vi "DequeueMessage.vi"(8 "error in (no error)":errorcluster, 9 "ms timeout (-1)":i32=-1, 11 "queue in":refnum<data-value>) -> (0 "error out":errorcluster, 1 "timeout":bool, 2 "message":variant, 3 "queue out":refnum<data-value>)   [LabVIEW 2009, in "PriorityQueue.lvclass"]
uses:
  PriorityQueue.lvclass
  LinkedList/position.ctl
  PriorityQueue.lvclass/PriorityQueue.ctl
  Message/Message.lvclass
  LLNode/LLNode.lvclass
  LinkedList/LinkedList.lvclass
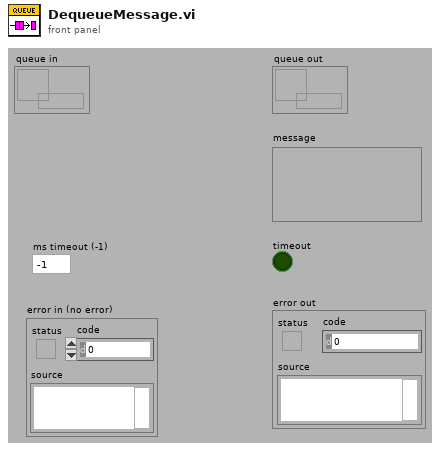
[diagram p1: front panel]
types:
  T1 = typedef "LinkedList.lvclass/position.ctl" = enum16{"Front", "Back", "Search"}
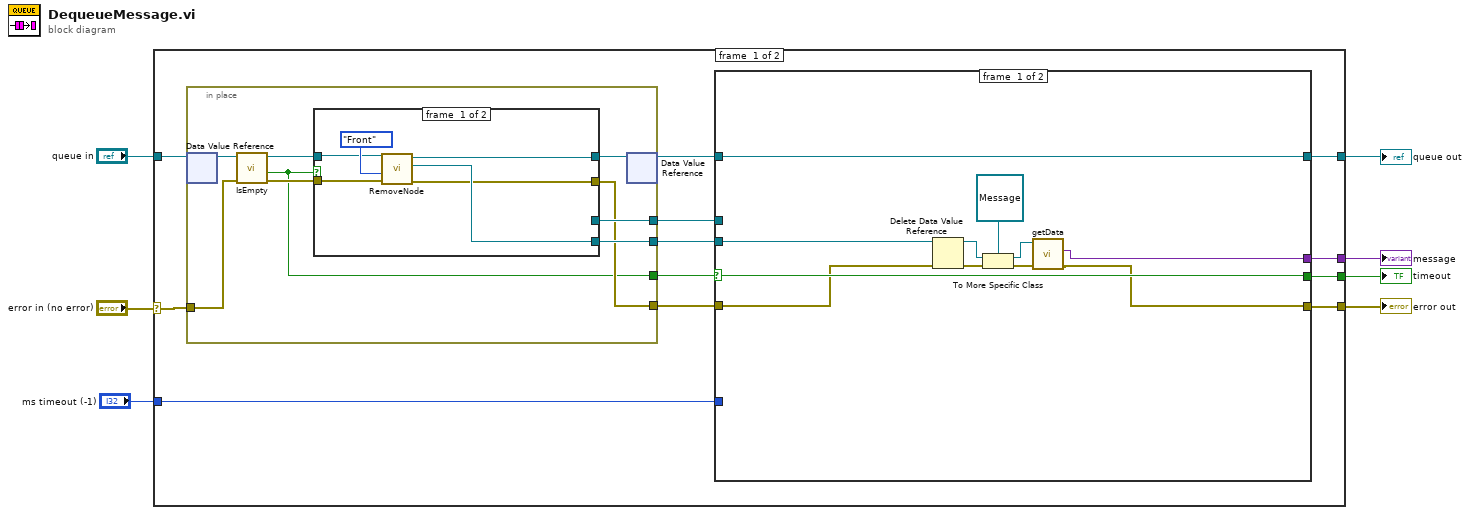
[diagram p0: block diagram]
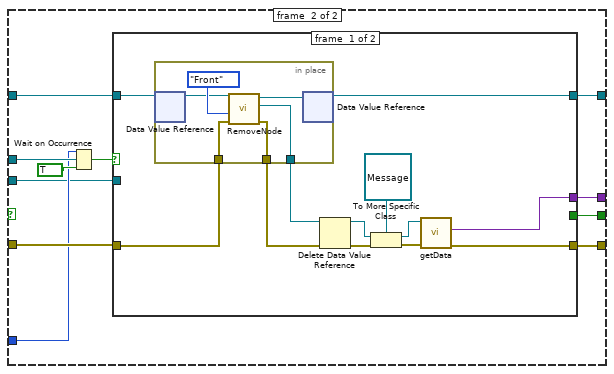
[diagram p2: hidden frame]
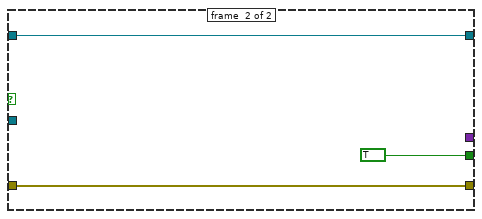
[diagram p3: hidden frame]
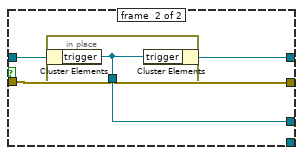
[diagram p4: hidden frame]
diagram:
  n1 = case shown="No Error" "error in (no error)" {
    selector: "error in (no error)" -> [w18 w83]
    tunnel: "queue in" -> [w19 w84]
    tunnel: [w17 w83] -> w6
    tunnel: [w14 _] -> w5
    tunnel: [w16 w84] -> w4
    tunnel: "ms timeout (-1)" -> [w8 _]
    tunnel: [w15 _] -> w1
    frame #0 {
      n2 = in-place {
        in-place-border: w18 -> [w70]
        in-place-border: [w67] -> w10
        in-place-border: [w65] -> w11
        in-place-border: [w64] -> w12
        in-place-border: [w63] -> w13
        n3 = in-place-dvr #1(w19) -> (w71:refnum<class "PriorityQueue.lvclass">)  [unwired: 1 out]
        n4 = call "IsEmpty.vi"("error in (no error)"=w70, "LinkedList in"=w71) -> ("error out"=w66:errorcluster, "empty"=w63:bool, "LinkedList out"=w69:refnum<class "PriorityQueue.lvclass">)  [unwired: 7 in]
        n5 = case shown="False" w63 {
          tunnel: w69 -> [w76 w81]
          tunnel: [w75 w80] -> w68
          tunnel: [_ w79] -> w67
          tunnel: w66 -> [w74 w78]
          tunnel: [w73 _] -> w65
          tunnel: [w72 w78] -> w64
          frame #0 {
            n6 = call "RemoveNode.vi"("error in (no error)"=w74, "position"=position."Front", "LinkedList in"=w76) -> ("error out"=w72:errorcluster, "RemovedNode"=w73:refnum<data-value>, "LinkedList out"=w75:refnum<class "PriorityQueue.lvclass">)  [unwired: 5 in, 1 out]
          }
          frame #1 {
            n7 = in-place {
              in-place-border: [w82] -> w79
              n8 = in-place-cluster #2(w81) -> ("trigger"=w82:refnum<k4>)
              n9 = in-place-cluster #2("trigger"=w82) -> (w80:refnum<class "PriorityQueue.lvclass">)
            }
          }
        }
        n10 = in-place-dvr #1(w68) -> (w9:refnum<data-value>)  [unwired: 1 out]
      }
      n11 = case shown="False" w13 {
        selector: w13 -> [w29 _]
        tunnel: w9 -> [w30 w41]
        tunnel: w12 -> [w28 w40]
        tunnel: [w20 w39] -> w17
        tunnel: [w30 w38] -> w16
        tunnel: [w21 w37] -> w15
        tunnel: [w29 w32] -> w14
        tunnel: w11 -> [w27 w31]
        tunnel: w10 -> [_ w36]
        tunnel: w8 -> [_ w34]
        frame #0 {
          n12 = Delete Data Value Reference(data value reference=w27, error in=w28) -> (data value=w22:refnum<class "LLNode.lvclass">, error out=w23:errorcluster)
          n13 = To More Specific Class(target class=refnum<class "Message.lvclass"> refnum ("Message out"), reference=w22, error in=w23) -> (specific class reference=w26:refnum<class "Message.lvclass">, error out=w24:errorcluster)
          n14 = call "getData.vi"("error in (no error)"=w24, "Message in"=w26) -> ("error out"=w20:errorcluster, "Data"=w21:variant)  [unwired: 7 in, 1 out]
        }
        frame #1 {
          n15 = Wait on Occurrence(1:TRUE ("ignore previous (T)"), 2:w36, 3:w34) -> (0:w33:bool)
          n16 = case shown="False" w33 {
            tunnel: w41 -> [w53 w61]
            tunnel: w40 -> [w52 w60]
            tunnel: [w47 w60] -> w39
            tunnel: [w51 w61] -> w38
            tunnel: [w50 _] -> w37
            tunnel: [_ TRUE] -> w32
            tunnel: w31 -> [_ _]
            frame #0 {
              n17 = in-place {
                in-place-border: w52 -> [w58]
                in-place-border: [w55] -> w49
                in-place-border: [w54] -> w48
                n18 = in-place-dvr #3(w53) -> (w57:refnum<class "PriorityQueue.lvclass">)  [unwired: 1 out]
                n19 = call "RemoveNode.vi"("error in (no error)"=w58, "position"=position."Front", "LinkedList in"=w57) -> ("error out"=w54:errorcluster, "RemovedNode"=w55:refnum<data-value>, "LinkedList out"=w56:refnum<class "PriorityQueue.lvclass">)  [unwired: 5 in, 1 out]
                n20 = in-place-dvr #3(w56) -> (w51:refnum<data-value>)  [unwired: 1 out]
              }
              n21 = Delete Data Value Reference(data value reference=w49, error in=w48) -> (data value=w45:refnum<class "LLNode.lvclass">, error out=w46:errorcluster)
              n22 = To More Specific Class(target class=refnum<class "Message.lvclass"> refnum ("Message out"), reference=w45, error in=w46) -> (specific class reference=w44:refnum<class "Message.lvclass">, error out=w42:errorcluster)
              n23 = call "getData.vi"("error in (no error)"=w42, "Message in"=w44) -> ("error out"=w47:errorcluster, "Data"=w50:variant)  [unwired: 7 in, 1 out]
            }
            frame #1 {
            }
          }
        }
      }
    }
    frame #1 {
    }
  }
  "queue out" <- w4
  "error out" <- w6
  "timeout" <- w5
  "message" <- w1
